vi "Tourner_Gyros.vi"(8 "Right":dbl, 9 "Left":dbl, 11 "Angle Voulu":dbl) -> (2 "Angle Reel":dbl)   [LabVIEW 2015]
uses:
  <vilib>/Rock Robotics/Network Tables/NT Write Number.vi
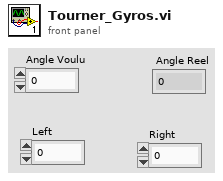
[diagram p1: front panel]
types:
  T1 = typedef "WPI_GyroDevRef.ctl" = cluster{"DevStatus":errorcluster, "Analog Channel":T2, "Offset":dbl, "Gain (VoltsPerDegree/Second)":dbl, "Gyro Type":enum16{"Analog", "XRS450"}, "Handle":i32, "SPI Bus":T3, "Device Found":bool, "Sample Rate":dbl, "Calibrate On Open":bool}
  T2 = typedef "FPGA_AIChannel.ctl" = enum8{"AI 0", "AI 1", "AI 2", "AI 3", "AI MXP 0", "AI MXP 1", "AI MXP 2", "AI MXP 3", "Invalid"}
  T3 = typedef "spi_bus.ctl" = enum16{"SPI On-Board, CS0", "SPI On-Board, CS1", "SPI On-Board, CS2", "SPI On-Board, CS3", "SPI MXP", "Invalid"}
  T4 = typedef "WPI_RobotDriveDevRef.ctl" = cluster{"DevStatus":errorcluster, "Motors[]":T5[], "Square Inputs":bool, "Max Output":dbl}
  T5 = typedef "WPI_MotorControlDeviceRef.ctl" = cluster{"DeviceStatus":errorcluster, "Type":T6, "PWM":cluster{"PWM Channel":T7, "DeadBand":T8}, "CAN":cluster{"Device Number":u8, "Control Mode":T9, "Semaphore":T10, "Max Vout":dbl, "TalonSRX Control Mode":T11}, "Invert":bool}
  T6 = typedef "WPI_MotorControlType.ctl" = enum16{"PWM", "CAN", "CANTalonSRX"}
  T7 = typedef "FPGA_DIOPWMChannel.ctl" = enum8{"PWM 0", "PWM 1", "PWM 2", "PWM 3", "PWM 4", "PWM 5", "PWM 6", "PWM 7", "PWM 8", "PWM 9", "PWM MXP 0", "PWM MXP 1", "PWM MXP 2", "PWM MXP 3", "PWM MXP 4", "PWM MXP 5", "PWM MXP 6", "PWM MXP 7", "PWM MXP 8", "PWM MXP 9", "Invalid"}
  T8 = typedef "WPI_PWMDeadband.ctl" = cluster{"Name":string, "maxPositivePwm":i32, "minPositivePwm":i32, "centerPwm":i32, "maxNegativePwm":i32, "minNegativePwm":i32, "angularRange":u16}
  T9 = typedef "WPI_CANJaguar_ControlMode.ctl" = enum8{"Percent VBus", "Current", "Speed", "Position", "Voltage"}
  T10 = typedef "Semaphore RefNum" = refnum<k1>
  T11 = typedef "WPI_CANTalonSRX_APIControlMode.ctl" = enum8{"Percent VBus", "Speed", "Position", "Slave", "Unchanged / Invalid", "Voltage Compensation", "Current", "Motion Profile"}
  T12 = typedef "WPI_EncoderDevRef.ctl" = cluster{"DevStatus":errorcluster, "EncoderIndex":T13, "CounterIndex":T14, "DistancePerCount":dbl, "Decoding Type":T15}
  T13 = typedef "FPGA_EncoderIdx.ctl" = enum8{"Enc 0", "Enc 1", "Enc 2", "Enc 3", "Enc 4", "Enc 5", "Enc 6", "Enc 7", "Invalid"}
  T14 = typedef "FPGA_CounterCtrSystemIndex.ctl" = enum8{"Ctr 0", "Ctr 1", "Ctr 2", "Ctr 3", "Ctr 4", "Ctr 5", "Ctr 6", "Ctr 7", "Invalid"}
  T15 = typedef "WPI_EncoderType.ctl" = enum16{"1x", "2x", "4x"}
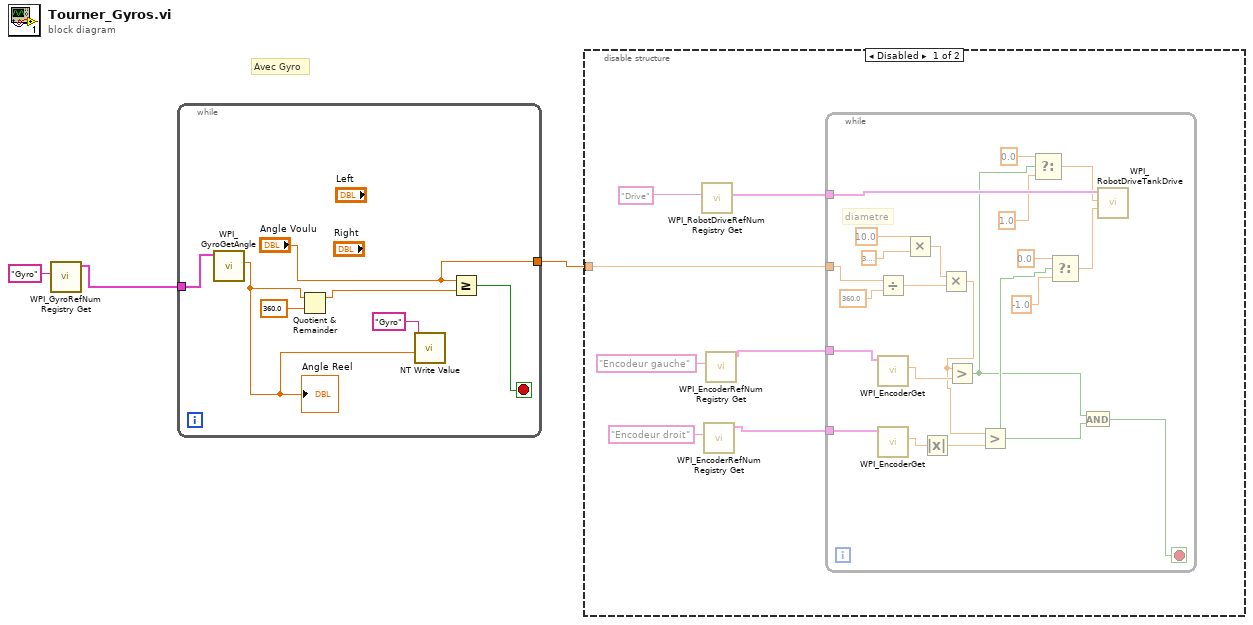
[diagram p0: block diagram]
diagram:
  # "Avec Gyro"
  n1 = call <vilib>:"WPI_GyroRefNum Registry Get.vi"("refnum name"="Gyro") -> ("GyroDevRef"=w3:T1)  [unwired: 9 in, 1 out]
  n2 = while {
    tunnel: w3 -> [w10]
    tunnel: ["Angle Voulu"] -> w1
    stop <- w9 stop-if-true
    n3 = call <vilib>:"WPI_GyroGetAngle.vi"("GyroDevRef"=w10) -> ("Angle"=w6:dbl)  [unwired: 6 in, 4 out]
    "Angle Reel" <- w6
    n4 = Quotient & Remainder(x=w6, y=360.0) -> (x-y*floor(x/y)=w7:dbl)  [unwired: 1 out]
    n5 = call-poly <vilib>:"NT Write Value.vi"("Numeric"=w6, "Name"="Gyro") -> ()  [unwired: 9 in, 1 out]
    n6 = Greater Or Equal?(x="Angle Voulu", y=w7) -> (x >= y?=w9:bool)
  }
  n7 = disable-structure shown="Disabled" {
    disable-tunnel: w1 -> [w11 _]
    frame Disabled {
      n8 = call <vilib>:"WPI_RobotDriveRefNum Registry Get.vi"("refnum name"="Drive") -> ("RobotDriveDevRef"=w16:T4)  [unwired: 9 in, 1 out]
      n9 = call <vilib>:"WPI_EncoderRefNum Registry Get.vi"("refnum name"="Encodeur droit") -> ("EncoderDevRef"=w15:T12)  [unwired: 9 in, 1 out]
      n10 = call <vilib>:"WPI_EncoderRefNum Registry Get.vi"("refnum name"="Encodeur gauche") -> ("EncoderDevRef"=w14:T12)  [unwired: 9 in, 1 out]
      n11 = while {
        tunnel: w16 -> [w39]
        tunnel: w15 -> [w38]
        tunnel: w14 -> [w37]
        tunnel: w11 -> [w36]
        stop <- w26 stop-if-true
        # "diametre"
        n12 = Divide(x=w36, y=360.0) -> (x/y=w34:dbl)
        n13 = call <vilib>:"WPI_EncoderGet.vi"("EncoderDevRef"=w37) -> ("Distance"=w30:dbl)  [unwired: 5 in, 5 out]
        n14 = call <vilib>:"WPI_EncoderGet.vi"("EncoderDevRef"=w38) -> ("Distance"=w28:dbl)  [unwired: 5 in, 5 out]
        n15 = Multiply(x=10.0, y=3.141592653589793) -> (x*y=w32:dbl)
        n16 = Absolute Value(x=w28) -> (abs(x)=w27:dbl)
        n17 = Multiply(x=w32, y=w34) -> (x*y=w29:dbl)
        n18 = Greater?(x=w29, y=w30) -> (0:w19:bool)
        n19 = Greater?(x=w29, y=w27) -> (0:w23:bool)
        n20 = Select(t=0.0, s=w19, f=1.0 ("Left axis value")) -> (s? t:f=w18:dbl)
        n21 = Select(t=0.0, s=w23, f=-1.0 ("Right axis value")) -> (s? t:f=w22:dbl)
        n22 = And(x=w19, y=w23) -> (x .and. y?=w26:bool)
        n23 = call <vilib>:"WPI_RobotDriveTankDrive.vi"("Right axis value"=w22, "Left axis value"=w18, "RobotDriveDevRef"=w39) -> ()  [unwired: 6 in, 3 out]
      }
    }
    frame Enabled {
    }
  }
